vi "TCP_Listener.vi"() -> ()   [LabVIEW 2019, in "Common System Tests.lvclass"]
uses:
  Common System Tests.lvclass
panel:
  out "No of messages":i32
  out "Recieved Messages":string[](array[string])
  out "current data out":string
  in  "error in (no error)":errorcluster
  out "error out":errorcluster
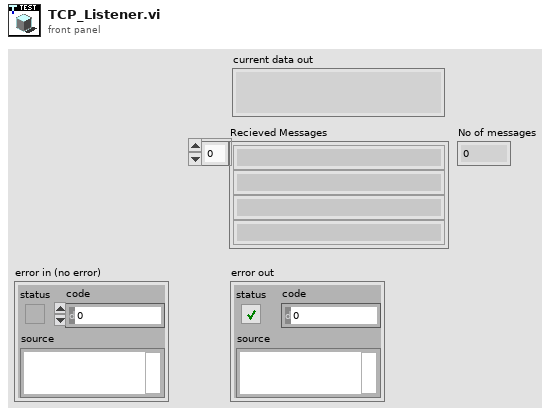
[diagram p1: front panel]
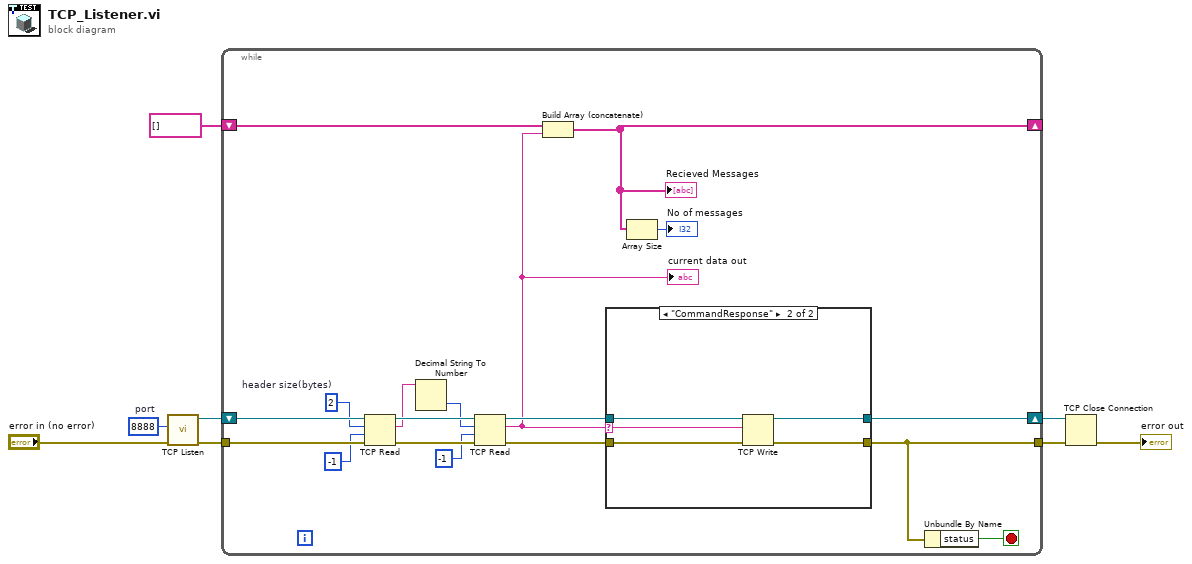
[diagram p0: block diagram]
diagram:
  w5 = u16 8888  # port
  n1 = call <vilib>:"TCP Listen.vi"("error in (no error)"="error in (no error)", "port"=w5) -> ("error out"=w3:errorcluster, "connection ID"=w4:refnum<k5>)  [unwired: 5 in, 3 out]
  n2 = while {
    shift-right: [w9] -> _
    shift-left: string[] [] -> [w24]
    shift-right: [w12] -> w8
    shift-left: w4 -> [w26]
    tunnel: w3 -> [w25]
    tunnel: [w14] -> w7
    stop <- w15 stop-if-true
    w23 = 2  # header size(bytes)
    n3 = TCP Read(connection ID=w26, bytes to read=w23, error in (no error)=w25, 9:-1 ("timeout ms (25000)")) -> (connection ID out=w20:refnum<k5>, data out=w19:string, error out=w21:errorcluster)  [unwired: 1 in]
    n4 = Decimal String To Number(string=w19) -> (number=w18:i32)  [unwired: 2 in, 1 out]
    n5 = TCP Read(connection ID=w20, bytes to read=w18, error in (no error)=w21, 9:-1 ("timeout ms (25000)")) -> (connection ID out=w13:refnum<k5>, data out=w11:string, error out=w16:errorcluster)  [unwired: 1 in]
    "current data out" <- w11
    n6 = Build Array (concatenate)(w24, w11) -> (w9:string[])
    "Recieved Messages" <- w9
    n7 = case shown="\"CommandResponse\"" w11 {
      selector: w11 -> [_ w29]
      tunnel: w16 -> [w28 w33]
      tunnel: [w28 w32] -> w14
      tunnel: w13 -> [w27 w31]
      tunnel: [w27 w30] -> w12
      frame "CommandOnly", Default {
      }
      frame "CommandResponse" {
        n8 = TCP Write(connection ID=w31, data in=w29, error in (no error)=w33) -> (connection ID out=w30:refnum<k5>, error out=w32:errorcluster)  [unwired: 1 in, 1 out]
      }
    }
    n9 = Array Size(array=w9) -> (size(s)=→"No of messages":i32)
    n10 = Unbundle By Name(w14) -> ("status"=w15:bool)
  }
  n11 = TCP Close Connection(connection ID=w8, error in (no error)=w7) -> (error out=→"error out":errorcluster)  [unwired: 1 in, 1 out]
